vi "Post PV Data.vi"(7 "PV name":string, 8 "error in":errorcluster, 10 "PV Data in":refnum<class "PV Data.lvclass">, 11 "Source in":refnum<class "Source.lvclass">) -> (0 "error out":errorcluster, 3 "Source out":refnum<class "Source.lvclass">)   [LabVIEW 2020, in "PV Access.lvlib" / "PVA Server.lvlib" / "Source.lvclass"]
uses:
  Source.lvclass
  PV Data/PV Data/PV Data.lvclass
  PV Access.lvlib
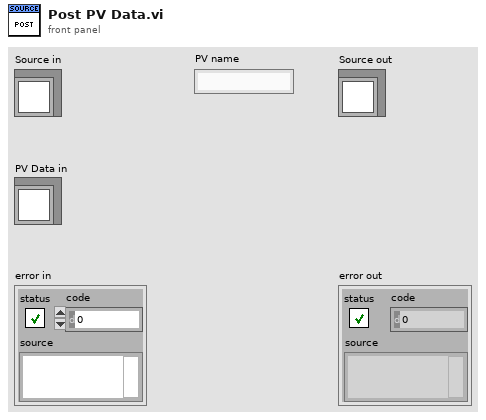
[diagram p1: front panel]
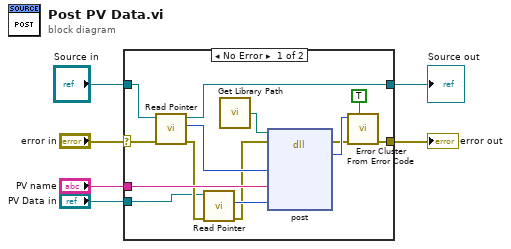
[diagram p0: block diagram]
diagram:
  n1 = case shown="No Error" "error in" {
    selector: "error in" -> [w20 w22]
    tunnel: [w7 w22] -> w5
    tunnel: [w16 w21] -> w1
    tunnel: "Source in" -> [w19 w21]
    tunnel: "PV name" -> [w15 _]
    tunnel: "PV Data in" -> [w11 _]
    frame No Error {
      n2 = call-dynamic "Read Pointer.vi"("error in (no error)"=w20, "Pointer Base in"=w19) -> ("error out"=w12:errorcluster, "Pointer"=w17:i64, "Pointer Base out"=w16:refnum<class "Source.lvclass">)  [unwired: 7 in]
      n3 = call-dynamic "Read Pointer.vi"("error in (no error)"=w12, "Pointer Base in"=w11) -> ("error out"=w13:errorcluster, "Pointer"=w14:i64)  [unwired: 7 in, 1 out]
      n4 = call "Get Library Path.vi"() -> ("Path"=w18:path)  [unwired: 1 in]
      n5 = dll-call lib="?" fn="post"(path in=w18, error in=w13, "source"=w17, "pv_name"=w15, "value"=w14) -> (error out=w8:errorcluster, "err_code"=w9:i32)  [unwired: 4 in, 1 out]
      n6 = call <vilib>:"Error Cluster From Error Code.vi"("show call chain? (False)"=TRUE, "error in (no error)"=w8, "error code (0)"=w9) -> ("error out"=w7:errorcluster)  [unwired: 6 in]
    }
    frame Error {
    }
  }
  "error out" <- w5
  "Source out" <- w1
